vi "kill task and queues for flystart.vi"() -> ()   [LabVIEW 2012]
panel:
  out "error out 8":errorcluster
  out "error out 7":errorcluster
  out "error out 6":errorcluster
  out "error out 5":errorcluster
  out "error out 4":errorcluster
  out "error out 3":errorcluster
  out "error out 2":errorcluster
  out "error out":errorcluster
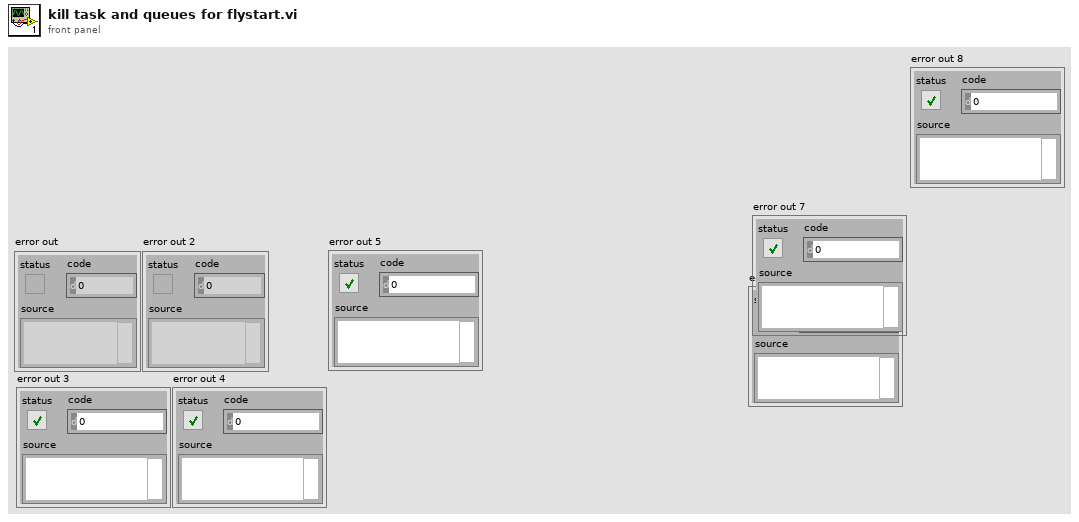
[diagram p1: front panel]
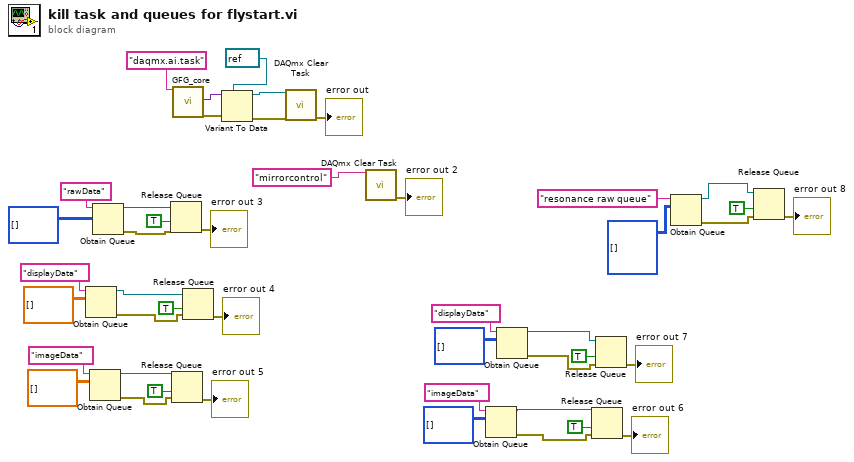
[diagram p0: block diagram]
diagram:
  n1 = Obtain Queue(name (unnamed)="displayData", element data type=dbl[][] [] ("y backward image")) -> (queue out=w34:refnum<queue>, error out=w20:errorcluster)  [unwired: 3 in, 1 out]
  n2 = Obtain Queue(name (unnamed)="imageData", element data type=dbl[][] [] ("y backward image")) -> (queue out=w30:refnum<queue>, error out=w21:errorcluster)  [unwired: 3 in, 1 out]
  n3 = Obtain Queue(name (unnamed)="rawData", element data type=i16[][] [] ("-x")) -> (queue out=w39:refnum<queue>, error out=w19:errorcluster)  [unwired: 3 in, 1 out]
  n4 = Release Queue(queue=w39, force destroy? (F)=TRUE, error in (no error)=w19) -> (error out=→"error out 3":errorcluster)  [unwired: 2 out]
  n5 = Release Queue(queue=w30, force destroy? (F)=TRUE, error in (no error)=w21) -> (error out=→"error out 5":errorcluster)  [unwired: 2 out]
  n6 = call "GFG_core.vi"("Variable Name in"="daqmx.ai.task") -> ("Variant Out"=w43:variant, "error out"=w7:errorcluster)  [unwired: 12 in, 5 out]
  n7 = Release Queue(queue=w34, force destroy? (F)=TRUE, error in (no error)=w20) -> (error out=→"error out 4":errorcluster)  [unwired: 2 out]
  n8 = Variant To Data(error in=w7, type=refnum<k21> refnum ("task out"), Variant=w43) -> (data=w45:refnum<k21>, error out=w8:errorcluster)
  n9 = call <vilib>:"DAQmx Clear Task.vi"("task in"=w45, "error in"=w8) -> ("error out"=→"error out":errorcluster)  [unwired: 13 in]
  n10 = call <vilib>:"DAQmx Clear Task.vi"("task in"="mirrorcontrol" ("name to assign")) -> ("error out"=→"error out 2":errorcluster)  [unwired: 14 in]
  n11 = Obtain Queue(name (unnamed)="imageData", element data type=i16[][] [] ("y backward image")) -> (queue out=w16:refnum<queue>, error out=w15:errorcluster)  [unwired: 3 in, 1 out]
  n12 = Obtain Queue(name (unnamed)="displayData", element data type=i16[][] [] ("y backward image")) -> (queue out=w9:refnum<queue>, error out=w10:errorcluster)  [unwired: 3 in, 1 out]
  n13 = Release Queue(queue=w16, force destroy? (F)=TRUE, error in (no error)=w15) -> (error out=→"error out 6":errorcluster)  [unwired: 2 out]
  n14 = Release Queue(queue=w9, force destroy? (F)=TRUE, error in (no error)=w10) -> (error out=→"error out 7":errorcluster)  [unwired: 2 out]
  n15 = Obtain Queue(name (unnamed)="resonance raw queue", element data type=i32[][][] [] ("initialized array")) -> (queue out=w1:refnum<queue>, error out=w2:errorcluster)  [unwired: 3 in, 1 out]
  n16 = Release Queue(queue=w1, force destroy? (F)=TRUE, error in (no error)=w2) -> (error out=→"error out 8":errorcluster)  [unwired: 2 out]
